vi "Day 4.2 - .vi"(11 "input":string[](array[string])) -> (3 "output":i16)   [LabVIEW 2021]
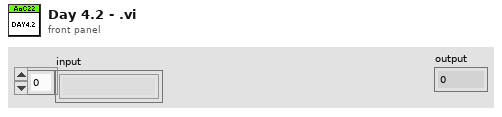
[diagram p1: front panel]
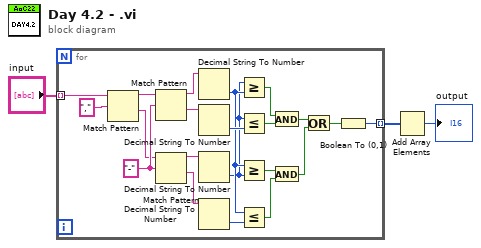
[diagram p0: block diagram]
diagram:
  n1 = for {
    tunnel: "input" -> [w17] mode=indexing
    tunnel: [w18] -> w2 mode=indexing
    w23 = "-" ("regular expression")
    n2 = Match Pattern(string=w17, regular expression=",") -> (before substring=w16:string, after substring=w15:string)  [unwired: 1 in, 2 out]
    n3 = Match Pattern(string=w16, regular expression=w23) -> (before substring=w22:string, after substring=w21:string)  [unwired: 1 in, 2 out]
    n4 = Match Pattern(string=w15, regular expression=w23) -> (before substring=w20:string, after substring=w19:string)  [unwired: 1 in, 2 out]
    n5 = Decimal String To Number(string=w22) -> (number=w9:i32)  [unwired: 2 in, 1 out]
    n6 = Decimal String To Number(string=w21) -> (number=w12:i32)  [unwired: 2 in, 1 out]
    n7 = Decimal String To Number(string=w20) -> (number=w4:i32)  [unwired: 2 in, 1 out]
    n8 = Decimal String To Number(string=w19) -> (number=w8:i32)  [unwired: 2 in, 1 out]
    n9 = Greater Or Equal?(x=w4, y=w9) -> (x >= y?=w13:bool)
    n10 = Less Or Equal?(x=w4, y=w12) -> (x <= y?=w14:bool)
    n11 = Greater Or Equal?(x=w9, y=w4) -> (x >= y?=w7:bool)
    n12 = Less Or Equal?(x=w9, y=w8) -> (x <= y?=w6:bool)
    n13 = And(x=w13, y=w14) -> (x .and. y?=w11:bool)
    n14 = And(x=w7, y=w6) -> (x .and. y?=w5:bool)
    n15 = Or(x=w11, y=w5) -> (x .or. y?=w10:bool)
    n16 = Boolean To (0,1)(Boolean=w10) -> (0, 1=w18:i16)
  }
  n17 = Add Array Elements(numeric array=w2) -> (sum=→"output":i16)
